vi "2-2.vi"() -> ()   [LabVIEW 2022 SP3]
panel:
  in  "确定按钮":bool
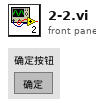
[diagram p1: front panel]
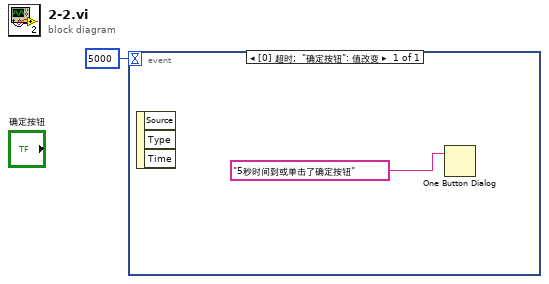
[diagram p0: block diagram]
diagram:
  n1 = event shown="[0] 超时;  \"确定按钮\": 值改变" {
    selector: _ -> [_]
    dyn-events: _ -> [_]
    timeout: 5000 -> [_]
    event Timeout; "确定按钮": Value Change {
      n2 = event-data() -> ()  [unwired: 1 in, 3 out]
      n3 = One Button Dialog(message="5秒时间到或单击了确定按钮" ("按钮名称（“确定”）")) -> ()  [unwired: 1 in, 1 out]
    }
  }
